vi "Intake Controller.vi"(8 "error in":errorcluster) -> ()   [LabVIEW 2017]
doc: "This VI executes continuously carrying out the current operation and responding to updates or new operations. It will often contain the timing or control code that is difficult to place directly in TeleOp. This VI generally opens all sensors and motors and isolates the rest of the robot code from knowing how the operations are carried out."
uses:
  <vilib>/Rock Robotics/WPI/Framework/Completion Status.ctl
  Intake Setpoints.ctl
  Intake Operations.ctl
  <vilib>/Rock Robotics/WPI/ThirdParty/Phoenix-LabVIEW/Motor Controller/Controls/CTRE_Phoenix_MotorControl_ControlMode.ctl
  <vilib>/Rock Robotics/WPI/ThirdParty/Phoenix-LabVIEW/Motor Controller/Get/CTRE_Phoenix_MotorController_GetOutputCurrent_Enhanced.vi
  <vilib>/Rock Robotics/Network Tables/NT Write Numeric Array.vi
panel:
  out "Left":dbl(graph)=0.125
  out "Left 2":dbl=0.125
  out "Right":dbl(graph)=0.125
  out "Right 2":dbl=0.125
  in  "Interactive Values":T1
  out "Current\nCmd":string
  in  "Buttons":cluster{"Execute Cmd":bool, "Abort Cmd":bool}
  out "Command Timing":cluster{"Start Time (ms)":u32, "Iterations":i32}
  out "Status":T3
  # "Interactive Command: You may fill in the settings for a command\nand schedule it with the Execute button. You can observe and abort\nany command while fine tuning the code for the controller."
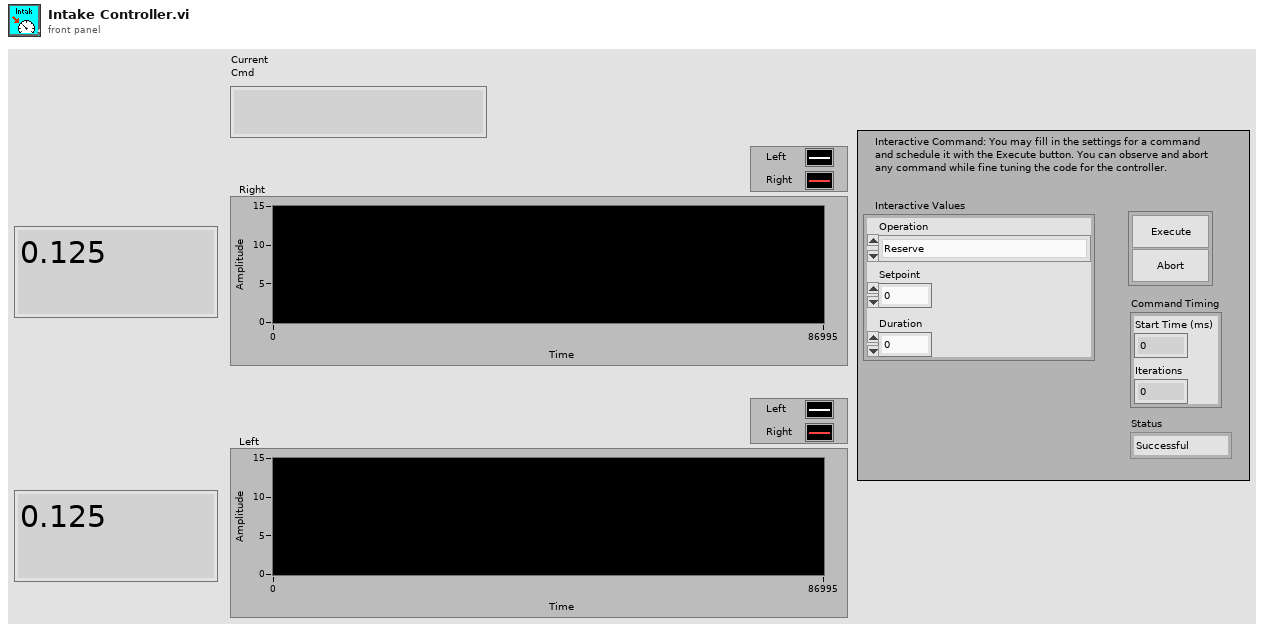
[diagram p1: front panel]
types:
  T1 = typedef "Intake Setpoints.ctl" = cluster{"Operation":T2, "Setpoint":dbl, "Duration":dbl}
  T2 = typedef "Intake Operations.ctl" = enum16{"Reserve", "Read Current", "Immediate", "Intake", "Eject", "Stop"}
  T3 = typedef "Completion Status.ctl" = enum16{"Successful", "Aborted", "Incomplete"}
  T4 = typedef "WPI_MotorControlDeviceRef.ctl" = cluster{"DeviceStatus":errorcluster, "Type":T5, "PWM":cluster{"PWM Channel":T6, "DeadBand":T7}, "CAN":cluster{"Device Number":u8, "SetOutput VI Ref":variant, "GetOutput VI Ref":variant, "Enable VI Ref":variant, "Disable VI Ref":variant, "Data":variant}, "Invert":bool, "DIO PWM":cluster{"PWM \"Enable\" Channel":T6, "DIOChannel":T8, "PWM Rate":dbl}}
  T5 = typedef "WPI_MotorControlType.ctl" = enum16{"PWM", "CAN", "DIO PWM"}
  T6 = typedef "FPGA_DIOPWMChannel.ctl" = enum8{"PWM 0", "PWM 1", "PWM 2", "PWM 3", "PWM 4", "PWM 5", "PWM 6", "PWM 7", "PWM 8", "PWM 9", "PWM MXP 0", "PWM MXP 1", "PWM MXP 2", "PWM MXP 3", "PWM MXP 4", "PWM MXP 5", "PWM MXP 6", "PWM MXP 7", "PWM MXP 8", "PWM MXP 9", "Invalid"}
  T7 = typedef "WPI_PWMDeadband.ctl" = cluster{"Name":string, "maxPositivePwm":i32, "minPositivePwm":i32, "centerPwm":i32, "maxNegativePwm":i32, "minNegativePwm":i32, "angularRange":u16}
  T8 = typedef "FPGA_DIOChannel.ctl" = enum8{"DIO 0", "DIO 1", "DIO 2", "DIO 3", "DIO 4", "DIO 5", "DIO 6", "DIO 7", "DIO 8", "DIO 9", "DIO MXP 0", "DIO MXP 1", "DIO MXP 2", "DIO MXP 3", "DIO MXP 4", "DIO MXP 5", "DIO MXP 6", "DIO MXP 7", "DIO MXP 8", "DIO MXP 9", "DIO MXP 10", "DIO MXP 11", "DIO MXP 12", "DIO MXP 13", "DIO MXP 14", "DIO MXP 15", "SPI Port CS1", "SPI Port CS2", "SPI Port CS3", "SPI Port MISO", "SPI Port MOSI", "Invalid"}
  T9 = typedef "Command Status Info.ctl" = cluster{"Name":string, "Status":T3, "notifier out":T10}
  T10 = typedef "Completion Notifier.ctl" = refnum<notifier>
  T11 = cluster{"Current Command":T1, "Command Timing":cluster{"Start Time (ms)":u32, "Iterations":i32}, "Command Arguments":cluster{"Command Info":T9, "Description":string, "Default Command":T1, "queue out":refnum<queue>, "Subsystem Name":string}}
  T12 = typedef "CTRE_Phoenix_MotorControl_ControlMode.ctl" = u16
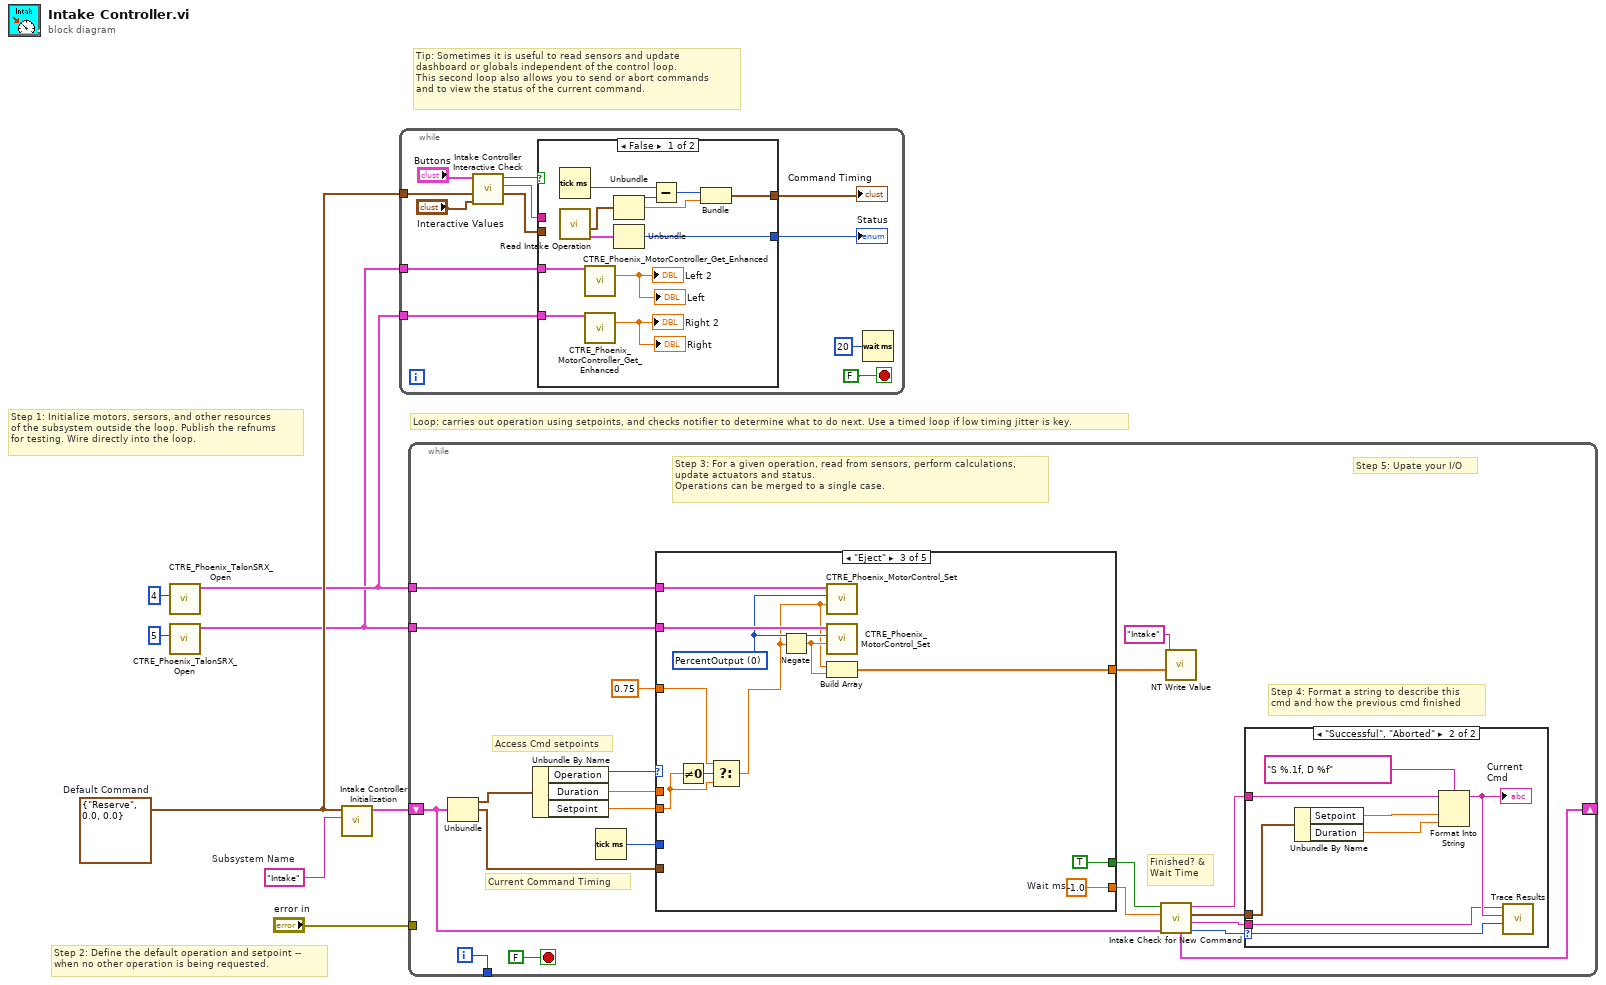
[diagram p0: block diagram]
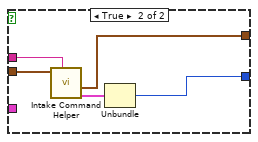
[diagram p2: hidden frame]
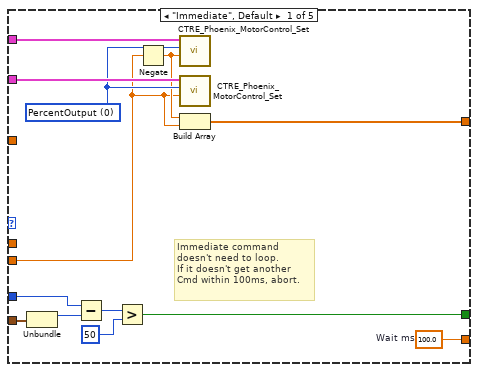
[diagram p4: hidden frame]
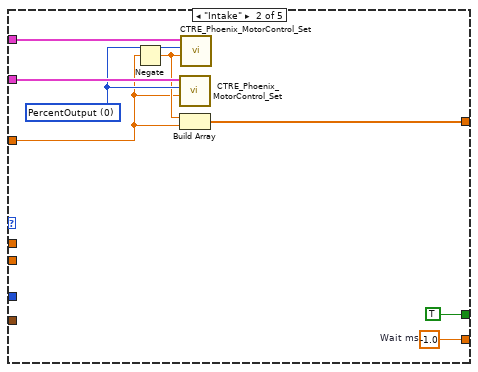
[diagram p5: hidden frame]
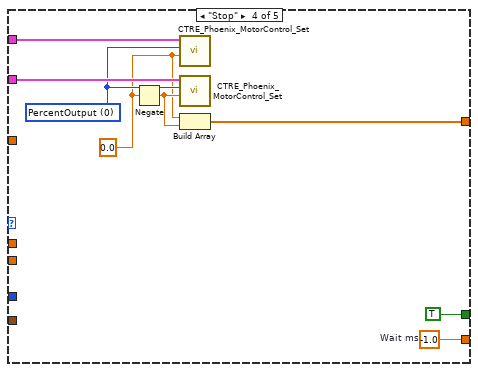
[diagram p6: hidden frame]
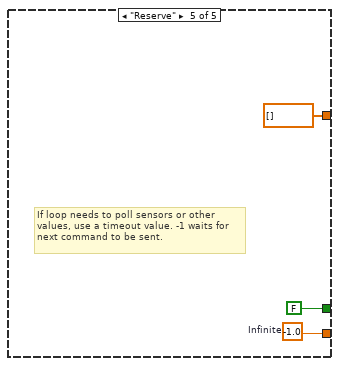
[diagram p7: hidden frame]
diagram:
  w5 = T1 {"Operation"=enum."Reserve", "Setpoint"=0.0, "Duration"=0.0}  # Default Command
  w6 = "Intake"  # Subsystem Name
  # "Tip: Sometimes it is useful to read sensors and update\ndashboard or globals independent of the control loop.\nThis second loop also allows you to send or abort commands\nand to view the status of the current command."
  # "Step 2: Define the default operation and setpoint --\nwhen no other operation is being requested."
  # "Step 1: Initialize motors, sersors, and other resources\nof the subsystem outside the loop. Publish the refnums\nfor testing. Wire directly into the loop."
  # "Loop: carries out operation using setpoints, and checks notifier to determine what to do next. Use a timed loop if low timing jitter is key."
  n1 = call <vilib>:"CTRE_Phoenix_TalonSRX_Open.vi"("Device Number"=u8 4) -> ("CAN Talon SRX Ref"=w2:T4)  [unwired: 9 in, 1 out]
  n2 = call <vilib>:"CTRE_Phoenix_TalonSRX_Open.vi"("Device Number"=u8 5) -> ("CAN Talon SRX Ref"=w1:T4)  [unwired: 9 in, 1 out]
  n3 = call "Intake Controller Initialization.vi"("Subsystem Name"=w6, "Default Command"=w5) -> ("Current Command"=w7:T11)  [unwired: 9 in]
  n4 = while {
    tunnel: w5 -> [w17]
    tunnel: w2 -> [w10]
    tunnel: w1 -> [w9]
    stop <- FALSE stop-if-true
    n5 = call "Intake Controller Interactive Check.vi"("Interactive Command in"="Interactive Values", "Default Command"=w17, "Buttons"="Buttons") -> ("Interactive Command out"=w14:T1, "Trace String"=w15:string, "Schedule"=w16:bool)  [unwired: 6 in]
    n6 = case shown="False" w16 {
      tunnel: [w32 w37] -> w13
      tunnel: w14 -> [_ w35]
      tunnel: [w28 w33] -> w12
      tunnel: w15 -> [_ w36]
      tunnel: w10 -> [w22 _]
      tunnel: w9 -> [w21 _]
      frame False {
        n7 = Tick Count (ms)() -> (millisecond timer value=w27:u32)
        n8 = call "Read Intake Operation.vi"() -> ("Command Info"=w25:T9, "SubSystem Data"=w26:T1)  [unwired: 9 in, 1 out]
        n9 = call-poly <vilib>:"CTRE_Phoenix_MotorController_Get_Enhanced.vi"("PhoenixMotorControlDevRef"=w21) -> ("Output Current"=→"Left 2" →"Left":dbl)  [unwired: 12 in, 2 out]
        n10 = call-poly <vilib>:"CTRE_Phoenix_MotorController_Get_Enhanced.vi"("PhoenixMotorControlDevRef"=w22) -> ("Output Current"=→"Right 2" →"Right":dbl)  [unwired: 12 in, 2 out]
        n11 = Unbundle(w26) -> ("Operation"=w31:T2, "Setpoint"=w29:dbl)  [unwired: 1 out]
        n12 = Unbundle(w25) -> ("Status"=w32:T3)  [unwired: 2 out]
        n13 = Subtract(x=w27, y=w31) -> (x-y=w30:u32)
        n14 = Bundle(w30, "Setpoint"=w29) -> (w28:cluster{u32, "Setpoint":dbl})  [unwired: 1 in]
      }
      frame True {
        n15 = call "Intake Command Helper.vi"("Description"=w36, "SubSystem Data"=w35) -> ("Command Info Out"=w34:T9, "Command Timing"=w33:cluster{"Start Time (ms)":u32, "Iterations":i32})  [unwired: 7 in, 1 out]
        n16 = Unbundle(w34) -> ("Status"=w37:T3)  [unwired: 2 out]
      }
    }
    "Status" <- w13
    "Command Timing" <- w12
    n17 = Wait (ms)(milliseconds to wait=u32 20) -> ()  [unwired: 1 out]
  }
  n18 = while {
    shift-right: [w50] -> _
    shift-left: w7 -> [w43]
    tunnel: [w57] -> _
    tunnel: "error in" -> [_]
    tunnel: w2 -> [w42]
    tunnel: w1 -> [w41]
    i -> [w57]
    stop <- FALSE stop-if-true
    # "Step 5: Upate your I/O"
    # "Step 4: Format a string to describe this\ncmd and how the previous cmd finished"
    # "Current Command Timing"
    # "Access Cmd setpoints"
    # "Finished? &\nWait Time"
    # "Step 3: For a given operation, read from sensors, perform calculations,\nupdate actuators and status.\nOperations can be merged to a single case."
    n19 = Unbundle(w43) -> ("Current Command"=w56:T1, "Command Timing"=w52:cluster{"Start Time (ms)":u32, "Iterations":i32})  [unwired: 1 out]
    n20 = Unbundle By Name(w56) -> ("Operation"=w55:T2, "Duration"=w54:dbl, "Setpoint"=w51:dbl)
    n21 = Tick Count (ms)() -> (millisecond timer value=w53:u32)
    n22 = case shown="\"Eject\"" w55 {
      tunnel: [w79 w87 w98 w106 w109] -> w48
      tunnel: [w73 TRUE ("ignore previous (F)") TRUE ("ignore previous (F)") TRUE ("ignore previous (F)") FALSE ("ignore previous (F)")] -> w49
      tunnel: w52 -> [w75 _ _ _ _]
      tunnel: w54 -> [_ _ _ _ _]
      tunnel: w53 -> [w74 _ _ _ _]
      tunnel: w51 -> [w67 _ w90 _ _]
      tunnel: w42 -> [w72 w86 w97 w105 _]
      tunnel: w41 -> [w71 w85 w96 w104 _]
      tunnel: [w69 w83 w94 w102 dbl[] []] -> w40
      tunnel: 0.75 ("Setpoint") -> [_ w80 w89 _ _]
      frame "Immediate", Default {
        w70 = T12 0 items=["PercentOutput"=0, "Position"=1, "Velocity"=2, "Current"=3, "Follower"=5, "MotionProfile"=6, "MotionMagic"=7, "MotionMagicArc"=8, "MotionProfileArc"=10, "Disabled"=15] ("Control Mode")
        w79 = 100.0  # Wait ms
        # "Immediate command\ndoesn't need to loop.\nIf it doesn't get another\nCmd within 100ms, abort."
        n23 = Unbundle(w75) -> ("Start Time (ms)"=w78:u32)  [unwired: 1 out]
        n24 = Subtract(x=w74, y=w78) -> (x-y=w77:u32)
        n25 = Greater?(x=w77, y=u8 50 ("Left Motor")) -> (0:w73:bool)
        n26 = Negate(x=w67) -> (-x=w68:dbl)
        n27 = call <vilib>:"CTRE_Phoenix_MotorControl_Set.vi"("Output"=w68, "Control Mode"=w70, "PhoenixMotorControlDevRef"=w72) -> ()  [unwired: 7 in, 2 out]
        n28 = call <vilib>:"CTRE_Phoenix_MotorControl_Set.vi"("Output"=w67, "Control Mode"=w70, "PhoenixMotorControlDevRef"=w71) -> ()  [unwired: 7 in, 2 out]
        n29 = Build Array(w68, w67) -> (w69:dbl[])
      }
      frame "Intake" {
        w84 = T12 0 items=["PercentOutput"=0, "Position"=1, "Velocity"=2, "Current"=3, "Follower"=5, "MotionProfile"=6, "MotionMagic"=7, "MotionMagicArc"=8, "MotionProfileArc"=10, "Disabled"=15] ("Control Mode")
        w87 = -1.0  # Wait ms
        n30 = Negate(x=w80) -> (-x=w81:dbl)
        n31 = call <vilib>:"CTRE_Phoenix_MotorControl_Set.vi"("Output"=w80, "Control Mode"=w84, "PhoenixMotorControlDevRef"=w85) -> ()  [unwired: 7 in, 2 out]
        n32 = Build Array(w81, w80) -> (w83:dbl[])
        n33 = call <vilib>:"CTRE_Phoenix_MotorControl_Set.vi"("Output"=w81, "Control Mode"=w84, "PhoenixMotorControlDevRef"=w86) -> ()  [unwired: 7 in, 2 out]
      }
      frame "Eject" {
        w95 = T12 0 items=["PercentOutput"=0, "Position"=1, "Velocity"=2, "Current"=3, "Follower"=5, "MotionProfile"=6, "MotionMagic"=7, "MotionMagicArc"=8, "MotionProfileArc"=10, "Disabled"=15] ("Control Mode")
        w98 = -1.0  # Wait ms
        n34 = Not Equal To 0?(x=w90) -> (x != 0?=w91:bool)
        n35 = Select(t=w89, s=w91, f=w90) -> (s? t:f=w88:dbl)
        n36 = Negate(x=w88) -> (-x=w92:dbl)
        n37 = call <vilib>:"CTRE_Phoenix_MotorControl_Set.vi"("Output"=w88, "Control Mode"=w95, "PhoenixMotorControlDevRef"=w97) -> ()  [unwired: 7 in, 2 out]
        n38 = call <vilib>:"CTRE_Phoenix_MotorControl_Set.vi"("Output"=w92, "Control Mode"=w95, "PhoenixMotorControlDevRef"=w96) -> ()  [unwired: 7 in, 2 out]
        n39 = Build Array(w88, w92) -> (w94:dbl[])
      }
      frame "Stop" {
        w99 = 0.0 ("Setpoint")
        w103 = T12 0 items=["PercentOutput"=0, "Position"=1, "Velocity"=2, "Current"=3, "Follower"=5, "MotionProfile"=6, "MotionMagic"=7, "MotionMagicArc"=8, "MotionProfileArc"=10, "Disabled"=15] ("Control Mode")
        w106 = -1.0  # Wait ms
        n40 = Negate(x=w99) -> (-x=w100:dbl)
        n41 = call <vilib>:"CTRE_Phoenix_MotorControl_Set.vi"("Output"=w99, "Control Mode"=w103, "PhoenixMotorControlDevRef"=w105) -> ()  [unwired: 7 in, 2 out]
        n42 = call <vilib>:"CTRE_Phoenix_MotorControl_Set.vi"("Output"=w100, "Control Mode"=w103, "PhoenixMotorControlDevRef"=w104) -> ()  [unwired: 7 in, 2 out]
        n43 = Build Array(w99, w100) -> (w102:dbl[])
      }
      frame "Reserve" {
        w109 = -1.0  # Infinite
        # "If loop needs to poll sensors or other\nvalues, use a timeout value. -1 waits for\nnext command to be sent."
      }
    }
    n44 = call "Intake Check for New Command.vi"("Current Command"=w43, "Wait time (ms)"=w48, "Finished?"=w49) -> ("Completion"=w44:T3, "Subsystem Name"=w45:string, "Current Command"=w46:T1, "Initial Trace String"=w47:string, "NextCommand"=w50:T11)  [unwired: 4 in]
    n45 = call-poly <vilib>:"NT Write Value.vi"("Numeric Array"=w40, "Name"="Intake") -> ()  [unwired: 9 in, 1 out]
    n46 = case shown="\"Successful\", \"Aborted\"" w44 {
      selector: w44 -> [_ w66]
      tunnel: w47 -> [_ w62]
      tunnel: w46 -> [_ w63]
      tunnel: w45 -> [_ w59]
      frame "Incomplete", Default {
        # "Continuing current command"
      }
      frame "Successful", "Aborted" {
        # "Report and setup for next command"
        n47 = Unbundle By Name(w63) -> ("Setpoint"=w65:dbl, "Duration"=w60:dbl)
        n48 = Format Into String(format string="S %.1f, D %f", initial string=w62, w65, w60) -> (resulting string=w61:string)  [unwired: 1 in, 1 out]
        "Current\nCmd" <- w61
        n49 = call <vilib>:"Trace Results.vi"("Status of previous command"=w66, "Description"=w61, "Subsystem"=w59) -> ()  [unwired: 9 in]
      }
    }
  }
